vi "CMWsubscribeINT(noinit).vi"(8 "error in":errorcluster, 11 "CMWintIN":refnum<class "CMWSubscribe.lvclass">) -> (0 "error out":errorcluster, 2 "CMWint":string, 3 "CMWintOUT":refnum<class "CMWSubscribe.lvclass">)   [LabVIEW 2014]
uses:
  <userlib>/_RADE/RIO/CMW/classes/CMWSubscribe/CMWSubscribe.lvclass
  <userlib>/_RADE/RIO/CMW/classes/CMWSubscribe/CMWSubscribe.vi
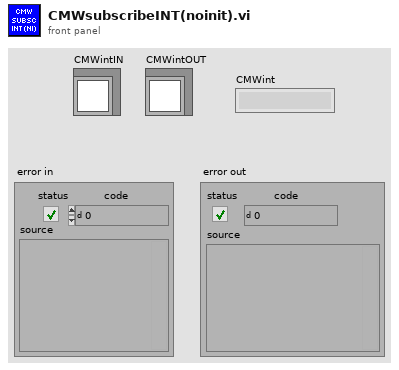
[diagram p1: front panel]
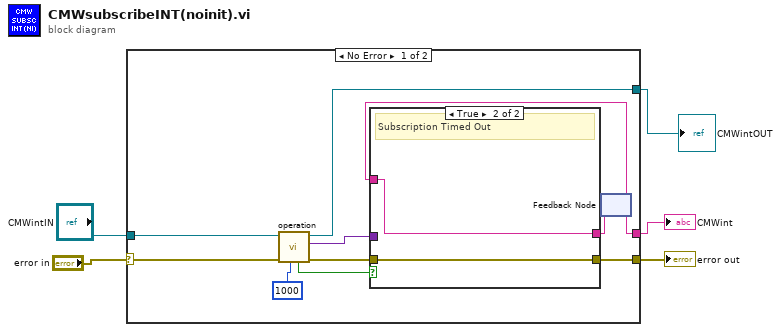
[diagram p0: block diagram]
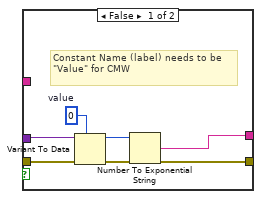
[diagram p2: hidden frame]
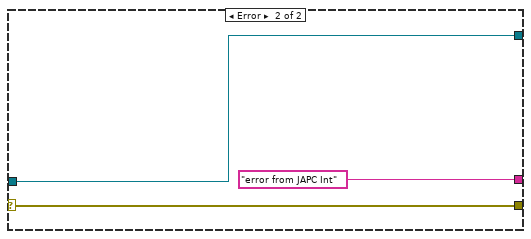
[diagram p3: hidden frame]
diagram:
  n1 = case shown="No Error" "error in" {
    selector: "error in" -> [w6 w26]
    tunnel: [w14 w26] -> w3
    tunnel: "CMWintIN" -> [w7 w25]
    tunnel: [w10 w25] -> w2
    tunnel: [w8 "error from JAPC Int"] -> w1
    frame No Error {
      n2 = call-poly <userlib>:"operation.vi"("Timeout (10000 ms)"=1000, "error in (no error)"=w6, "Object in"=w7) -> ("error out"=w15:errorcluster, "Data"=w11:variant, "Object out"=w10:refnum<class "CMWSubscribe.lvclass">, "Timeout?"=w12:bool)  [unwired: 4 in, 1 out]
      n3 = feedback #1() -> (w8:string)  [unwired: 1 in]
      n4 = case shown="True" w12 {
        tunnel: w15 -> [w21 w23]
        tunnel: [w19 w23] -> w14
        tunnel: w11 -> [w20 _]
        tunnel: [w17 w22] -> w9
        tunnel: w8 -> [_ w22]
        frame False {
          w16 = i16 0  # value
          # "Constant Name (label) needs to be \"Value\" for CMW"
          n5 = Variant To Data(error in=w21, type=w16, Variant=w20) -> (data=w18:i16, error out=w19:errorcluster)
          n6 = Number To Exponential String(number=w18) -> (E-format string=w17:string)  [unwired: 3 in]
        }
        frame True {
          # "Subscription Timed Out"
        }
      }
      n7 = feedback-in #1(w9) -> ()
    }
    frame Error {
    }
  }
  "error out" <- w3
  "CMWintOUT" <- w2
  "CMWint" <- w1
